vi "Initialize Attributes.vi"(8 "error in (no error)":errorcluster, 10 "Attribute Data":variant, 11 "CS++GoBangServer in":refnum<class "CS++GoBangServer.lvclass">) -> (0 "error out":errorcluster, 2 "Found?":bool, 3 "CS++GoBangServer out":refnum<class "CS++GoBangServer.lvclass">)   [LabVIEW 2014, in "GoBang.lvlib" / "CS++GoBangServer.lvclass"]
doc: "Initialize object attribute.\n\nUnique resources should be allocated elsewhere!"
uses:
  CS++GoBangServer.lvclass
  CSPP_Core/Classes/CS++ProcessVariables/SVConnection/SVConnection.lvclass
  CSPP_Core/Classes/CS++ProcessVariables/ProcessVariable/PV.lvclass
  CSPP_Core/Actors/CS++BaseActor/CS++BaseActor.lvclass/CS++BaseActor.ctl
  CSPP_Core/Classes/CS++ProcessVariables/ProcessVariable/PV.lvclass/PV.ctl
  CSPP_Core/Classes/CS++ProcessVariables/PVConnection/PVConnection.lvclass/PVConnection.ctl
  CS++GoBangServer.lvclass/CS++GoBangServer.ctl
  CSPP_Core/Actors/CS++BaseActor/CS++BaseActor.lvclass
  CSPP_Core/Classes/CS++BaseClasses/Factory/CS++Factory.lvclass
  CSPP_Core/Classes/CS++ProcessVariables/PVConnection/PVConnection.lvclass
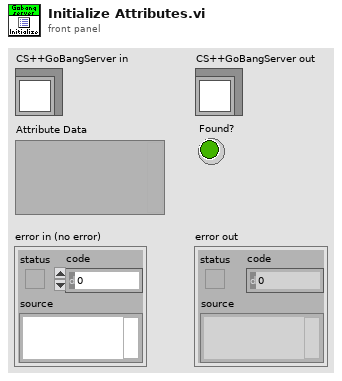
[diagram p1: front panel]
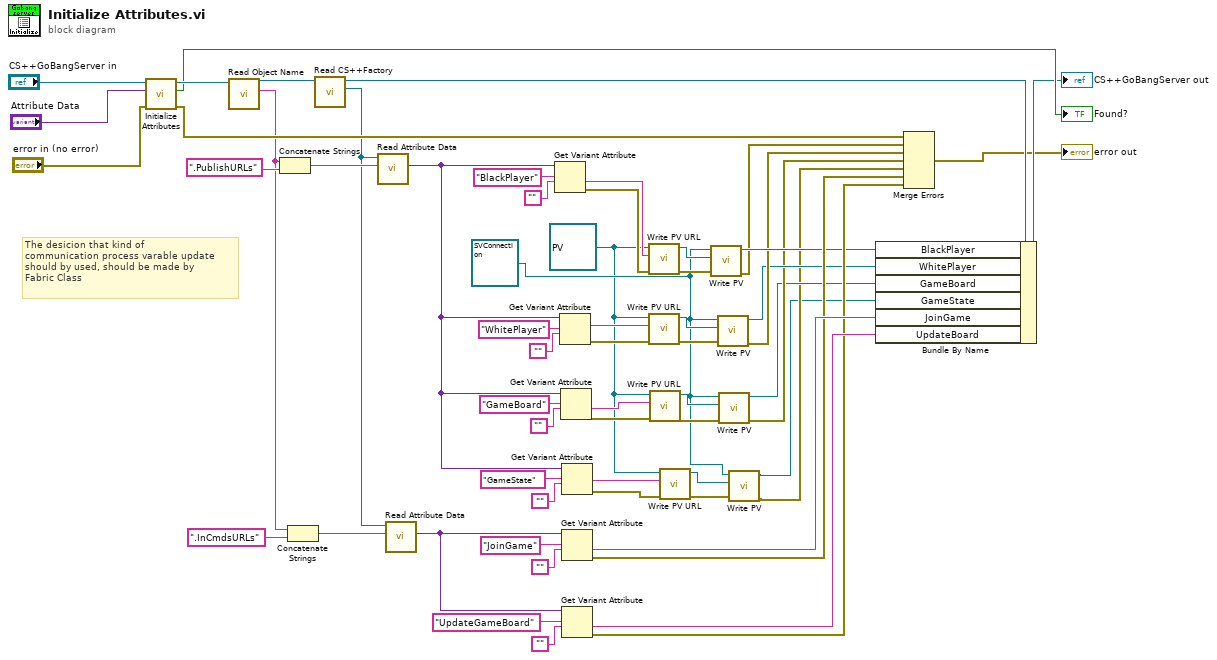
[diagram p0: block diagram]
diagram:
  w1 = refnum<class "PV.lvclass"> refnum ("CS++ProcessVariables.lvlib:PV.lvclass")
  w7 = refnum<class "SVConnection.lvclass"> refnum ("CS++ProcessVariables.lvlib:SVConnection.lvclass")
  # "The desicion that kind of\ncommunication process varable update \nshould by used, should be made by \nFabric Class"
  n1 = call-parent "Initialize Attributes.vi"("error in (no error)"="error in (no error)", "Attribute Data"="Attribute Data", "CS++BaseActor in"="CS++GoBangServer in") -> ("error out"=w60:errorcluster, "Found?"=→"Found?":bool, "CS++BaseActor out"=w55:refnum<class "CS++GoBangServer.lvclass">)  [unwired: 6 in]
  n2 = call "Read Object Name.vi"("CS++BaseActor in"=w55) -> ("Object Name"=w38:string, "CS++BaseActor out"=w56:refnum<class "CS++GoBangServer.lvclass">)  [unwired: 8 in, 1 out]
  n3 = Concatenate Strings(w38, ".PublishURLs" ("string")) -> (w51:string)
  n4 = Concatenate Strings(w38, ".InCmdsURLs" ("string")) -> (w39:string)
  n5 = call "Read CS++Factory.vi"("CS++BaseActor in"=w56) -> ("CS++Factory"=w35:refnum<class "CS++Factory.lvclass">, "CS++BaseActor out"=w54:refnum<class "CS++GoBangServer.lvclass">)  [unwired: 8 in, 1 out]
  n6 = call-dynamic "Read Attribute Data.vi"("Object Name"=w51, "CS++Factory in"=w35) -> ("Attribute Data"=w41:variant)  [unwired: 7 in, 2 out]
  n7 = call-dynamic "Read Attribute Data.vi"("Object Name"=w39, "CS++Factory in"=w35) -> ("Attribute Data"=w30:variant)  [unwired: 7 in, 2 out]
  n8 = Get Variant Attribute(Variant=w41, name="BlackPlayer", default value (empty Variant)="") -> (value=w26:string, error out=w23:errorcluster)  [unwired: 1 in, 2 out]
  n9 = Get Variant Attribute(Variant=w41, name="WhitePlayer", default value (empty Variant)="") -> (value=w19:string, error out=w18:errorcluster)  [unwired: 1 in, 2 out]
  n10 = Get Variant Attribute(Variant=w41, name="GameBoard", default value (empty Variant)="") -> (value=w9:string, error out=w13:errorcluster)  [unwired: 1 in, 2 out]
  n11 = Get Variant Attribute(Variant=w41, name="GameState", default value (empty Variant)="") -> (value=w2:string, error out=w6:errorcluster)  [unwired: 1 in, 2 out]
  n12 = Get Variant Attribute(Variant=w30, name="JoinGame", default value (empty Variant)="") -> (value=w33:string, error out=w28:errorcluster)  [unwired: 1 in, 2 out]
  n13 = Get Variant Attribute(Variant=w30, name="UpdateGameBoard", default value (empty Variant)="") -> (value=w29:string, error out=w27:errorcluster)  [unwired: 1 in, 2 out]
  n14 = call "Write PV URL.vi"("error in (no error)"=w23, "PV URL"=w26, "PV in"=w1) -> ("error out"=w22:errorcluster, "PV out"=w25:refnum<class "PV.lvclass">)  [unwired: 7 in]
  n15 = call "Write PV URL.vi"("error in (no error)"=w18, "PV URL"=w19, "PV in"=w1) -> ("error out"=w20:errorcluster, "PV out"=w15:refnum<class "PV.lvclass">)  [unwired: 7 in]
  n16 = call "Write PV URL.vi"("error in (no error)"=w13, "PV URL"=w9, "PV in"=w1) -> ("error out"=w11:errorcluster, "PV out"=w14:refnum<class "PV.lvclass">)  [unwired: 7 in]
  n17 = call "Write PV URL.vi"("error in (no error)"=w6, "PV URL"=w2, "PV in"=w1) -> ("error out"=w5:errorcluster, "PV out"=w8:refnum<class "PV.lvclass">)  [unwired: 7 in]
  n18 = call "Write PV.vi"("error in (no error)"=w22, "PV"=w25, "PVConnection in"=w7) -> ("error out"=w21:errorcluster, "PVConnection out"=w24:refnum<class "SVConnection.lvclass">)  [unwired: 7 in]
  n19 = call "Write PV.vi"("error in (no error)"=w20, "PV"=w15, "PVConnection in"=w7) -> ("error out"=w17:errorcluster, "PVConnection out"=w16:refnum<class "SVConnection.lvclass">)  [unwired: 7 in]
  n20 = call "Write PV.vi"("error in (no error)"=w11, "PV"=w14, "PVConnection in"=w7) -> ("error out"=w12:errorcluster, "PVConnection out"=w10:refnum<class "SVConnection.lvclass">)  [unwired: 7 in]
  n21 = call "Write PV.vi"("error in (no error)"=w5, "PV"=w8, "PVConnection in"=w7) -> ("error out"=w4:errorcluster, "PVConnection out"=w3:refnum<class "SVConnection.lvclass">)  [unwired: 7 in]
  n22 = Bundle By Name(cluster=w54, "BlackPlayer"=w24, "WhitePlayer"=w16, "GameBoard"=w10, "GameState"=w3, "JoinGame"=w33, "UpdateBoard"=w29) -> (→"CS++GoBangServer out":refnum<class "CS++GoBangServer.lvclass">)
  n23 = Merge Errors(w60, w21, w17, w12, w4, w28, w27) -> (→"error out":errorcluster)
